vi "DAQchannelStorage.vi"(2 "error in":errorcluster, 3 "Channel Settings":T1(array[cluster]), 4 "Tree DVR In":refnum<data-value>) -> (0 "error out":errorcluster)   [LabVIEW 2013]
uses:
  <vilib>/MDSplus/Classes/Tree_Class/Tree.lvclass
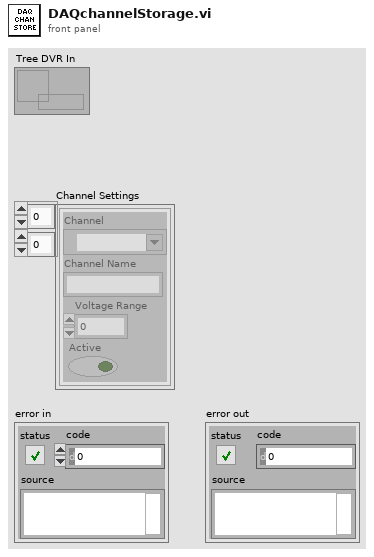
[diagram p1: front panel]
types:
  T1 = cluster{"Channel":tag, "Channel Name":string, "Voltage Range":dbl, "Active":bool}[][]
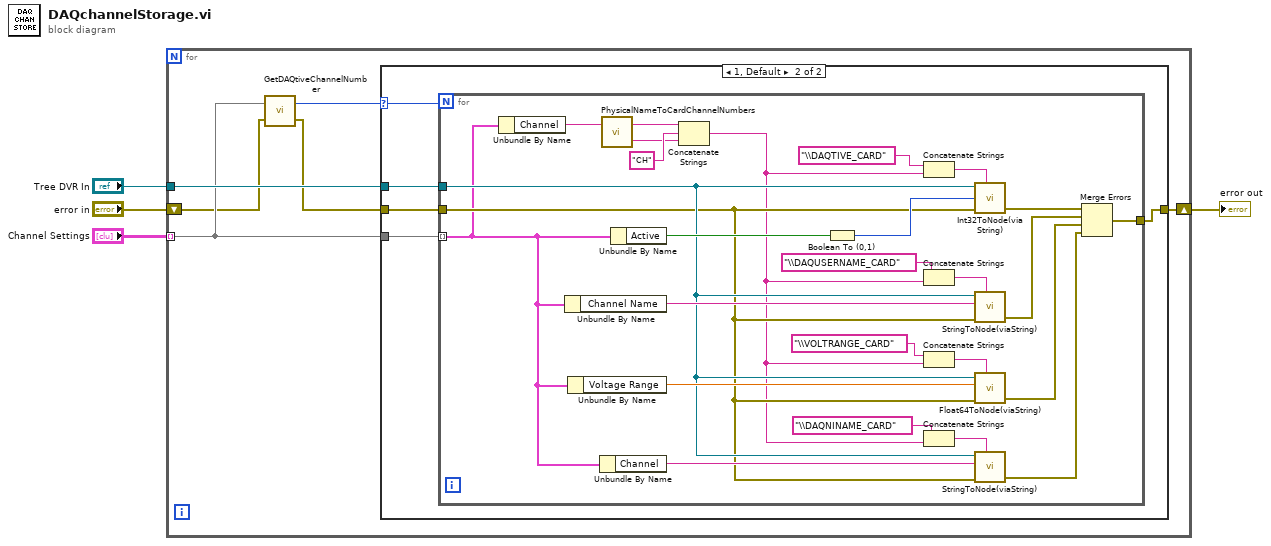
[diagram p0: block diagram]
diagram:
  n1 = for {
    shift-right: [w9] -> w1
    shift-left: "error in" -> [w6]
    tunnel: "Channel Settings" -> [w7] mode=indexing
    tunnel: "Tree DVR In" -> [w10]
    n2 = call "GetDAQtiveChannelNumber.vi"("error in (no error)"=w6, "Channel Settings"=w7) -> ("error out"=w5:errorcluster, "Numeric"=w8:i32)
    n3 = case shown="1, Default" w8 {
      selector: w8 -> [_ w12]
      tunnel: w7 -> [_ w16]
      tunnel: w5 -> [w11 w15]
      tunnel: w10 -> [_ w14]
      tunnel: [w11 w13] -> w9
      frame 0 {
      }
      frame 1, Default {
        n4 = for {
          N: w12 -> [_]
          tunnel: w16 -> [w23] mode=indexing
          tunnel: w15 -> [w29]
          tunnel: w14 -> [w30]
          tunnel: [w27] -> w13
          n5 = Unbundle By Name(w23) -> ("Channel"=w22:tag)
          n6 = Unbundle By Name(w23) -> ("Channel Name"=w37:string)
          n7 = Unbundle By Name(w23) -> ("Voltage Range"=w34:dbl)
          n8 = Unbundle By Name(w23) -> ("Channel"=w31:tag)
          n9 = call "PhysicalNameToCardChannelNumbers.vi"("NI Physical Channel"=w22) -> ("Channel #"=w24:string, "Card #"=w25:string)  [unwired: 1 in]
          n10 = Unbundle By Name(w23) -> ("Active"=w40:bool)
          n11 = Concatenate Strings(w25, "CH" ("string"), w24) -> (w18:string)
          n12 = Boolean To (0,1)(Boolean=w40) -> (0, 1=w42:i16)
          n13 = Concatenate Strings("\\DAQTIVE_CARD" ("string"), w18) -> (w41:string)
          n14 = Concatenate Strings("\\DAQUSERNAME_CARD" ("string"), w18) -> (w38:string)
          n15 = Concatenate Strings("\\VOLTRANGE_CARD" ("string"), w18) -> (w35:string)
          n16 = Concatenate Strings("\\DAQNINAME_CARD" ("string"), w18) -> (w32:string)
          n17 = call "Int32ToNode(viaString).vi"("Tree DVR in"=w30, "I32 in"=w42, "error in (no error)"=w29, "NodePath"=w41) -> ("error out"=w39:errorcluster)  [unwired: 1 in, 2 out]
          n18 = call "StringToNode(viaString).vi"("Tree DVR in"=w30, "String value in"=w37, "error in (no error)"=w29, "NodePath"=w38) -> ("error out"=w36:errorcluster)  [unwired: 1 in, 2 out]
          n19 = call "Float64ToNode(viaString).vi"("Tree DVR in"=w30, "DBL in"=w34, "error in"=w29, "NodePath"=w35) -> ("error out"=w33:errorcluster)  [unwired: 1 in, 2 out]
          n20 = call "StringToNode(viaString).vi"("Tree DVR in"=w30, "String value in"=w31, "error in (no error)"=w29, "NodePath"=w32) -> ("error out"=w28:errorcluster)  [unwired: 1 in, 2 out]
          n21 = Merge Errors(w39, w36, w33, w28) -> (w27:errorcluster)
        }
      }
    }
  }
  "error out" <- w1
